vi "To LabVIEW.vi"(4 "BB Players Map in":refnum<class "BB Players Map.lvclass">, 7 "ExpectedType":refnum<class>, 8 "error in (no error)":errorcluster, 10 "DbRow":variant) -> (0 "error out":errorcluster, 2 "Value":refnum<class>)   [LabVIEW 2020, in "BB Players Map.lvclass"]
doc: "This converts a \"DbRow\" structure, which is a set of name:value pairs implemented as variant attributes, into the private data for the bbPlayers class."
uses:
  BB Players Map.lvclass
  C:/Program Files/National Instruments/LabVIEW 2020/vi.lib/Viviota/shared/ORM.lvlibp/ORM/TypeMap/TypeMap.lvclass
  BB Players/bbPlayers.lvclass
  <vilib>/Viviota/shared/ORM.lvlibp/ORM/TypeMap/Read Autokey.vi
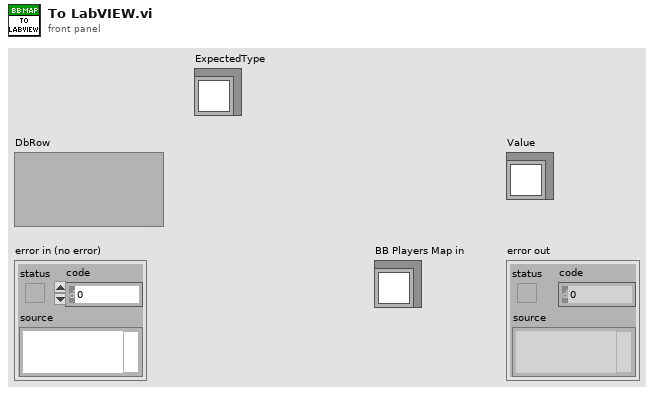
[diagram p1: front panel]
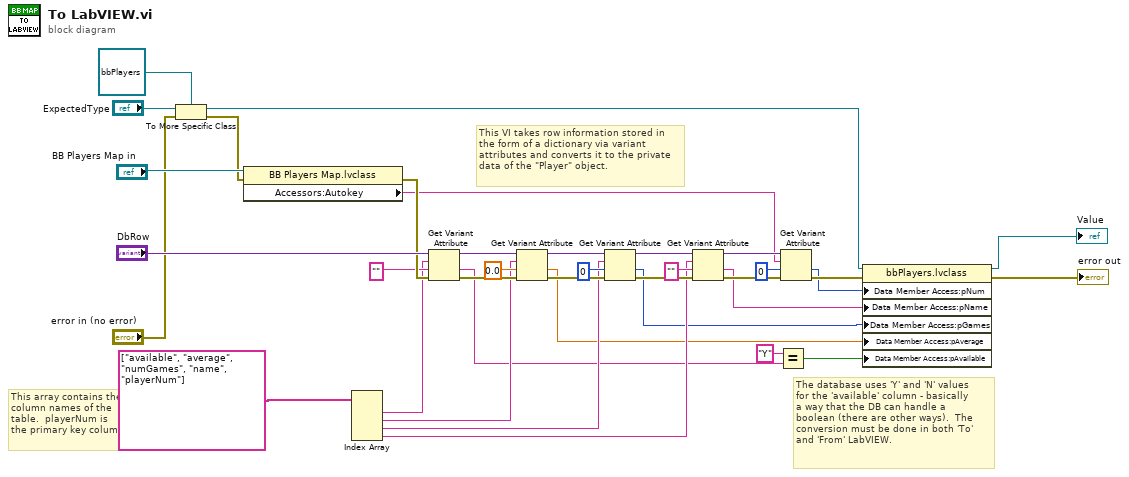
[diagram p0: block diagram]
diagram:
  # "The database uses 'Y' and 'N' values\nfor the 'available' column - basically \na way that the DB can handle a\nboolean (there are other ways).  The\nconversion must be done in both 'To'\nand 'From' LabVIEW."
  # "This array contains the\ncolumn names of the\ntable.  playerNum is\nthe primary key column."
  # "This VI takes row information stored in\nthe form of a dictionary via variant\nattributes and converts it to the private\ndata of the \"Player\" object."
  n1 = To More Specific Class(target class=refnum<class "bbPlayers.lvclass"> refnum ("bbPlayers.lvclass"), reference="ExpectedType", error in="error in (no error)") -> (specific class reference=w1:refnum<class "bbPlayers.lvclass">, error out=w3:errorcluster)
  n2 = property class="BB Players Map.lvclass"(reference="BB Players Map in", error in=w3) -> (error out=w35:errorcluster, "Accessors:Autokey"=w7:string)  [unwired: 1 out]
  n3 = Index Array(array=string[] ["available", "average", "numGames", "name", "playerNum"]) -> (element #1=w16:string, element #2=w15:string, element #3=w14:string, element #4=w13:string)  [unwired: 4 in]
  n4 = Get Variant Attribute(Variant="DbRow", name=w16, default value (empty Variant)="", error in=w35) -> (duplicate Variant=w30:variant, value=w12:string, error out=w34:errorcluster)  [unwired: 1 out]
  n5 = Get Variant Attribute(Variant=w30, name=w15, default value (empty Variant)=0.0, error in=w34) -> (duplicate Variant=w29:variant, value=w10:dbl, error out=w33:errorcluster)  [unwired: 1 out]
  n6 = Get Variant Attribute(Variant=w29, name=w14, default value (empty Variant)=0, error in=w33) -> (duplicate Variant=w28:variant, value=w9:i32, error out=w32:errorcluster)  [unwired: 1 out]
  n7 = Get Variant Attribute(Variant=w28, name=w13, default value (empty Variant)="", error in=w32) -> (duplicate Variant=w27:variant, value=w8:string, error out=w31:errorcluster)  [unwired: 1 out]
  n8 = Equal?(x="Y", y=w12) -> (x = y?=w11:bool)
  n9 = Get Variant Attribute(Variant=w27, name=w7, default value (empty Variant)=0, error in=w31) -> (value=w6:i32, error out=w25:errorcluster)  [unwired: 2 out]
  n10 = property class="bbPlayers.lvclass"(reference=w1, error in=w25, "Data Member Access:pNum"=w6, "Data Member Access:pName"=w8, "Data Member Access:pGames"=w9, "Data Member Access:pAverage"=w10, "Data Member Access:pAvailable"=w11) -> (reference out=→"Value":refnum<class "bbPlayers.lvclass">, error out=→"error out":errorcluster)
